vi "PWM.Measure.Analog.vi"(10 "PWM":fxp<+/-,32,8>, 11 "Settings":T3={"ACTIVE EDGE"=TRUE, "TIMEOUT"=40000000, "VMAX"=12.0, "THRESHOLD"=50.0}) -> (2 "Update?":bool, 3 "Measurement":T1)   [LabVIEW 2015, in "Speciality FPGA IO.lvlib"]
uses:
  Speciality FPGA IO.lvlib
  Types/PWM.Measure.Analog.Settings.ctl
  Types/PWM.Measure.Analog.Internal.ctl
  Types/PWM.Measure.Analog.Measurement.ctl
  <vilib>/rvi/Emulation/niFpgaSctlEmulationGetInTimedLoop.vi
  <vilib>/rvi/Emulation/niFpgaProcessEmulError.vi
panel:
  out "Local.State":bool
  out "Local.Data":T2
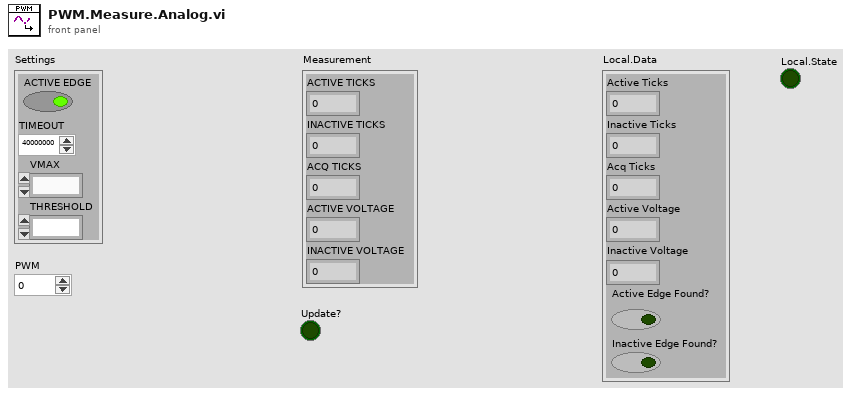
[diagram p1: front panel]
types:
  T1 = typedef "Speciality FPGA IO.lvlib/PWM.Measure.Analog.Measurement.ctl" = cluster{"ACTIVE TICKS":u32, "INACTIVE TICKS":u32, "ACQ TICKS":u32, "ACTIVE VOLTAGE":fxp<+/-,32,8>, "INACTIVE VOLTAGE":fxp<+/-,32,8>}
  T2 = typedef "Speciality FPGA IO.lvlib/PWM.Measure.Analog.Internal.ctl" = cluster{"Active Ticks":u32, "Inactive Ticks":u32, "Acq Ticks":u32, "Active Voltage":fxp<+/-,32,8>, "Inactive Voltage":fxp<+/-,32,8>, "Active Edge Found?":bool, "Inactive Edge Found?":bool}
  T3 = typedef "Speciality FPGA IO.lvlib/PWM.Measure.Analog.Settings.ctl" = cluster{"ACTIVE EDGE":bool, "TIMEOUT":u32, "VMAX":fxp<+/-,32,8>, "THRESHOLD":fxp<+,31,7>}
  T4 = enum8{"Initialize", "Wait on Active Edge", "Wait on Inactive Edge"}
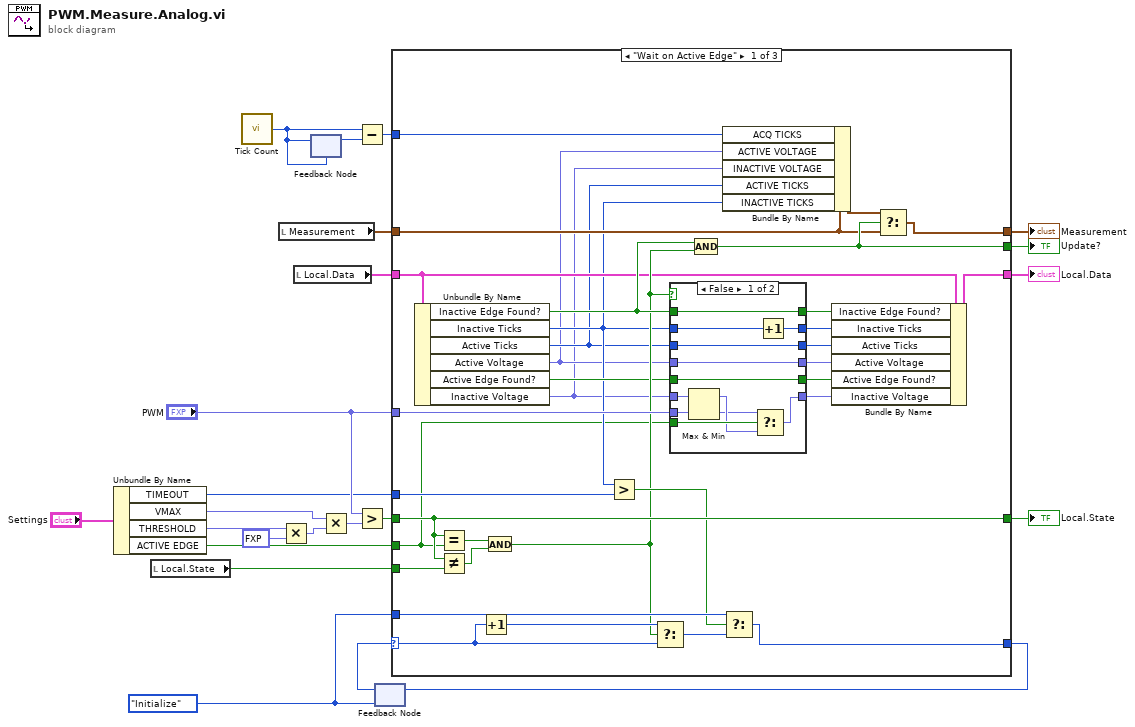
[diagram p0: block diagram]
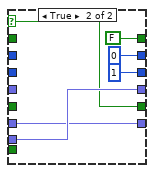
[diagram p2: hidden frame]
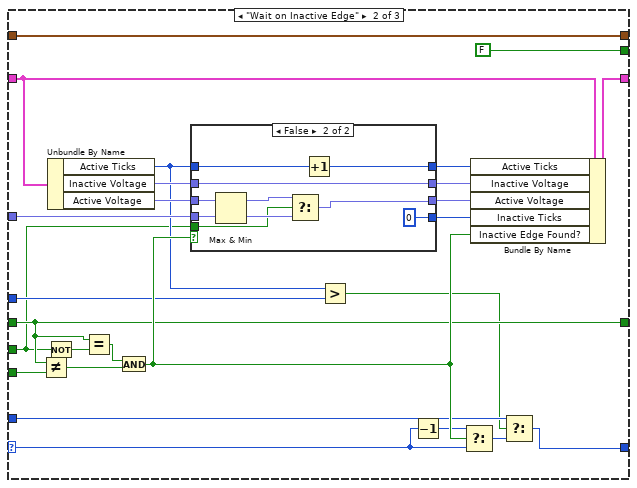
[diagram p3: hidden frame]
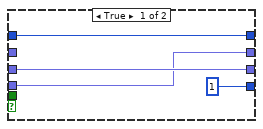
[diagram p4: hidden frame]
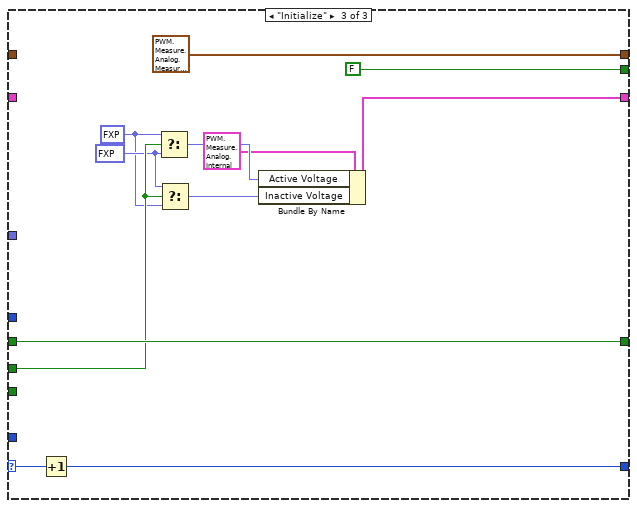
[diagram p5: hidden frame]
diagram:
  w10 = T4."Initialize"
  n1 = Unbundle By Name("Settings") -> ("TIMEOUT"=w2:u32, "VMAX"=w3:fxp<+/-,32,8>, "THRESHOLD"=w19:fxp<+,31,7>, "ACTIVE EDGE"=w16:bool)
  n2 = local read "Local.State"() -> (w14:bool)
  n3 = call "Tick Count"() -> ("Tick Count(Ticks)"=w7:u32)
  n4 = local read "Measurement"() -> (w12:T1)
  n5 = Multiply(x=w19, y=fxp<+,31,7> 0.009999990463256836) -> (x*y=w4:fxp<+,32,0>)
  n6 = local read "Local.Data"() -> (w20:T2)
  n7 = feedback-in #1(w7) -> ()
  n8 = feedback #1(w7) -> (w8:u32)
  n9 = Multiply(x=w3, y=w4) -> (x*y=w18:fxp<+/-,32,8>)
  n10 = Subtract(x=w7, y=w8) -> (x-y=w6:u32)
  n11 = Greater?(x="PWM", y=w18) -> (0:w17:bool)
  n12 = feedback #2(w10) -> (w22:T4)
  n13 = case shown="\"Wait on Active Edge\"" w22 {
    selector: w22 -> [w55 w84 w126]
    tunnel: [w53 w98 w118] -> w23
    tunnel: [w37 w77 w125] -> w21
    tunnel: w20 -> [w32 w97 _]
    tunnel: w17 -> [w45 w86 w124]
    tunnel: w16 -> [w24 w75 w123]
    tunnel: [w45 w86 w124] -> w15
    tunnel: w14 -> [w56 w100 _]
    tunnel: "PWM" -> [w47 w95 _]
    tunnel: [w48 w92 T1 {"ACTIVE TICKS"=0, "INACTIVE TICKS"=0, "ACQ TICKS"=0, "ACTIVE VOLTAGE"=0.0, "INACTIVE VOLTAGE"=0.0} ("Cached.Data")] -> w5
    tunnel: w12 -> [w29 w92 _]
    tunnel: w2 -> [w41 w81 _]
    tunnel: w10 -> [w40 w80 _]
    tunnel: [w36 FALSE FALSE] -> w9
    tunnel: w6 -> [w30 _ _]
    frame "Wait on Active Edge" {
      n14 = Unbundle By Name(w32) -> ("Inactive Edge Found?"=w49:bool, "Inactive Ticks"=w28:u32, "Active Ticks"=w27:u32, "Active Voltage"=w26:fxp<+/-,32,8>, "Active Edge Found?"=w33:bool, "Inactive Voltage"=w25:fxp<+/-,32,8>)
      n15 = Equal?(x=w45, y=w24) -> (x = y?=w44:bool)
      n16 = Not Equal?(x=w45, y=w56) -> (x != y?=w43:bool)
      n17 = Increment(x=w55) -> (x+1=w54:T4)
      n18 = And(x=w44, y=w43) -> (x .and. y?=w35:bool)
      n19 = Greater?(x=w28, y=w41) -> (0:w39:bool)
      n20 = Select(t=w54, s=w35, f=w55) -> (s? t:f=w38:T4)
      n21 = case shown="False" w35 {
        selector: w35 -> [_ w69]
        tunnel: [w57 w71] -> w52
        tunnel: [w67 u32 0 ("Inactive time")] -> w51
        tunnel: w28 -> [w68 _]
        tunnel: w25 -> [w66 w71]
        tunnel: w49 -> [w65 _]
        tunnel: [w65 FALSE ("Inactive Edge Found?")] -> w50
        tunnel: w47 -> [w64 w72]
        tunnel: [w63 w72] -> w46
        tunnel: w26 -> [w63 _]
        tunnel: [w62 u32 1 ("t")] -> w42
        tunnel: w27 -> [w62 _]
        tunnel: [w61 w69] -> w34
        tunnel: w33 -> [w61 _]
        tunnel: w24 -> [w60 _]
        frame False {
          n22 = Max & Min(x=w66, y=w64) -> (max(x,y)=w59:fxp<+/-,32,8>, min(x,y)=w58:fxp<+/-,32,8>)
          n23 = Select(t=w58, s=w60, f=w59) -> (s? t:f=w57:fxp<+/-,32,8>)
          n24 = Increment(x=w68) -> (x+1=w67:u32)
        }
        frame True {
        }
      }
      n25 = Compound Arithmetic op=AND(w49, w35) -> (w36:bool)
      n26 = Bundle By Name(cluster=w29, "ACQ TICKS"=w30, "ACTIVE VOLTAGE"=w26, "INACTIVE VOLTAGE"=w25, "ACTIVE TICKS"=w27, "INACTIVE TICKS"=w28) -> (w31:T1)
      n27 = Select(t=w40, s=w39, f=w38) -> (s? t:f=w37:T4)
      n28 = Bundle By Name(cluster=w32, "Inactive Edge Found?"=w50, "Inactive Ticks"=w51, "Active Ticks"=w42, "Active Voltage"=w46, "Active Edge Found?"=w34, "Inactive Voltage"=w52) -> (w53:T2)
      n29 = Select(t=w31, s=w36, f=w29) -> (s? t:f=w48:T1)
    }
    frame "Wait on Inactive Edge" {
      n30 = Not Equal?(x=w86, y=w100) -> (x != y?=w99:bool)
      n31 = Not(x=w75) -> (.not. x?=w87:bool)
      n32 = Unbundle By Name(w97) -> ("Active Ticks"=w82:u32, "Inactive Voltage"=w90:fxp<+/-,32,8>, "Active Voltage"=w96:fxp<+/-,32,8>)
      n33 = Equal?(x=w86, y=w87) -> (x = y?=w85:bool)
      n34 = And(x=w85, y=w99) -> (x .and. y?=w88:bool)
      n35 = case shown="False" w88 {
        tunnel: w96 -> [w103 w114]
        tunnel: w95 -> [w102 w113]
        tunnel: [w103 w106] -> w94
        tunnel: w82 -> [w104 w112]
        tunnel: [w104 w111] -> w93
        tunnel: [w102 w110] -> w91
        tunnel: w90 -> [_ w110]
        tunnel: [u32 1 ("t") u32 0 ("t")] -> w89
        tunnel: w75 -> [_ w105]
        frame True {
        }
        frame False {
          n36 = Max & Min(x=w114, y=w113) -> (max(x,y)=w107:fxp<+/-,32,8>, min(x,y)=w108:fxp<+/-,32,8>)
          n37 = Select(t=w107, s=w105, f=w108) -> (s? t:f=w106:fxp<+/-,32,8>)
          n38 = Increment(x=w112) -> (x+1=w111:u32)
        }
      }
      n39 = Greater?(x=w82, y=w81) -> (0:w79:bool)
      n40 = Decrement(x=w84) -> (x-1=w83:T4)
      n41 = Select(t=w83, s=w88, f=w84) -> (s? t:f=w78:T4)
      n42 = Bundle By Name(cluster=w97, "Active Ticks"=w93, "Inactive Voltage"=w91, "Active Voltage"=w94, "Inactive Ticks"=w89, "Inactive Edge Found?"=w88) -> (w98:T2)
      n43 = Select(t=w80, s=w79, f=w78) -> (s? t:f=w77:T4)
    }
    frame "Initialize" {
      w121 = fxp<+/-,32,8> -128.0 ("Active Voltage")
      w120 = fxp<+/-,32,8> 127.99998474121094 ("Active Voltage")
      n44 = Increment(x=w126) -> (x+1=w125:T4)
      n45 = Select(t=w120, s=w123, f=w121) -> (s? t:f=w122:fxp<+/-,32,8>)
      n46 = Select(t=w121, s=w123, f=w120) -> (s? t:f=w119:fxp<+/-,32,8>)
      n47 = Bundle By Name(cluster=T2 {"Active Ticks"=0, "Inactive Ticks"=0, "Acq Ticks"=0, "Active Voltage"=0.0, "Inactive Voltage"=0.0, "Active Edge Found?"=FALSE, "Inactive Edge Found?"=FALSE} ("Result"), "Active Voltage"=w122, "Inactive Voltage"=w119) -> (w118:T2)
    }
  }
  "Local.Data" <- w23
  "Local.State" <- w15
  "Measurement" <- w5
  "Update?" <- w9
  n48 = feedback-in #2(w21) -> ()
